vi "变更暂存.vi"(8 "error in":errorcluster caption="错误输入（无错误）", 10 "变更项":string[](array[string]), 11 "仓库路径":path=path "E:/学习文件/Git插件/test") -> (0 "error out":errorcluster caption="错误输出", 1 "standard error":string caption="标准错误", 2 "standard output":string caption="标准输出", 3 "仓库路径":path=path "E:/学习文件/Git插件/test")   [LabVIEW 2018]
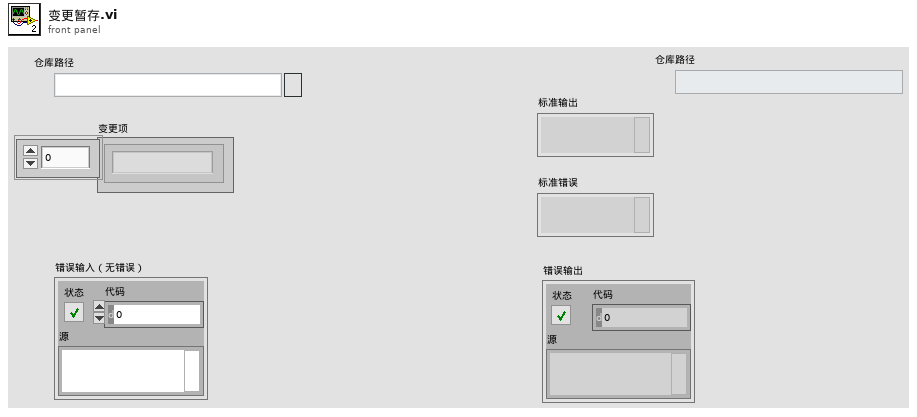
[diagram p1: front panel]
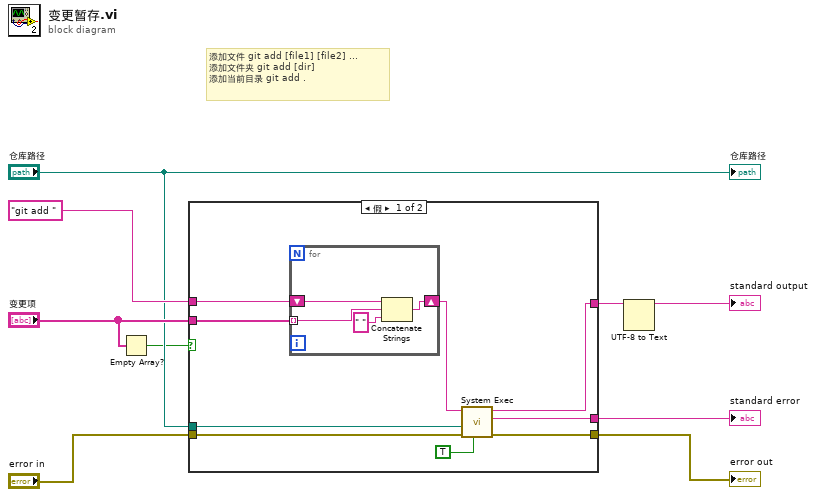
[diagram p0: block diagram]
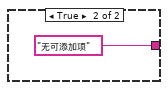
[diagram p2: hidden frame]
diagram:
  # "添加文件 git add [file1] [file2] ...\n添加文件夹 git add [dir]\n添加当前目录 git add ."
  n1 = Empty Array?(array="变更项") -> (empty?=w1:bool)
  n2 = case shown="假" w1 {
    tunnel: [w18 _] -> w9
    tunnel: [w17 "无可添加项" ("standard output")] -> w8
    tunnel: "变更项" -> [w15 _]
    tunnel: "git add " ("command line") -> [w14 _]
    tunnel: "error in" -> [w12 _]
    tunnel: [w11 _] -> w3
    tunnel: "仓库路径" -> [w10 _]
    frame False {
      n3 = for {
        tunnel: w15 -> [w22] mode=indexing
        shift-right: [w20] -> w13
        shift-left: w14 -> [w19]
        n4 = Concatenate Strings(w19, w22, " " ("字符串")) -> (w20:string)
      }
      n5 = call <vilib>:"System Exec.vi"("run minimized? (F)"=TRUE, "error in (no error)"=w12, "working directory"=w10, "command line"=w13) -> ("error out"=w11:errorcluster, "standard error"=w18:string, "standard output"=w17:string)  [unwired: 4 in, 1 out]
    }
    frame True {
    }
  }
  "standard error" <- w9
  "error out" <- w3
  n6 = UTF-8 to Text ("UTF-8至文本转换")(11:w8) -> (3:→"standard output":string)  [unwired: 2 in, 1 out]
  "仓库路径" <- "仓库路径"
